vi "Turn filter wheel by angle.vi"(8 "Clockwise?":bool=TRUE, 9 "Error In":errorcluster, 11 "Angle (degrees)":dbl=50.5244026184082) -> (0 "error out":errorcluster, 2 "Enable Channel out":u8=11, 3 "Serial Port out":refnum<visa-resource-name>="COM3")   [LabVIEW 2011]
uses:
  <vilib>/MakerHub/LINX/Public/Peripherals/Digital/Digital Write 1 Chan.vi
  <vilib>/MakerHub/LINX/LMH-LINX.lvlib
panel:
  in  "Enable Channel":u8=11
  in  "Direction Channel":u8=8
  in  "Step Channel":u8=9
  in  "Serial Port":refnum<visa-resource-name>="COM6"
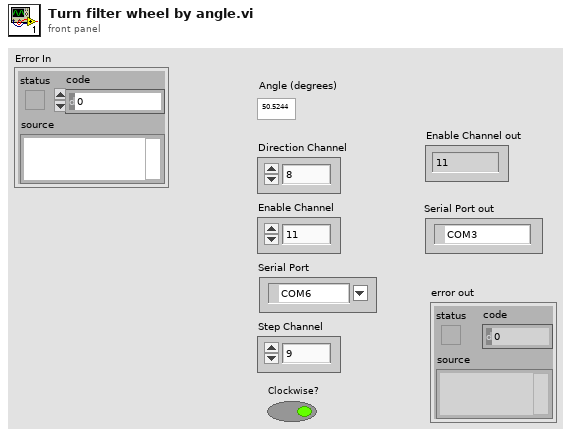
[diagram p1: front panel]
types:
  T1 = typedef "LMH-LINX.lvlib/LINX Ref.ctl" = cluster{"Platform":T2, "Interface":T3, "LINX Device Config":T4}
  T2 = typedef "LMH-LINX.lvlib/Platform.ctl" = enum16{"LINX", "myRIO"}
  T3 = typedef "LMH-LINX.lvlib/Interface.ctl" = enum16{"Serial", "TCP"}
  T4 = typedef "LMH-LINX.lvlib/Device.lvlib/LINX Device Config.ctl" = cluster{"Interface":T3, "COM Port":refnum<visa-resource-name>, "TCP Configuration":T5, "Device Family":u8, "Device ID":u8, "Device Name":string, "TCP Ref":refnum<k5>, "Channels":T6}
  T5 = typedef "LMH-LINX.lvlib/Device.lvlib/TCP Config.ctl" = cluster{"IP Address":string, "Port":u16}
  T6 = typedef "LMH-LINX.lvlib/Channels.ctl" = cluster{"DI":u8[], "DO":u8[], "AI":u8[], "AO":u8[], "PWM":u8[], "QE":u8[], "UART":u8[], "I2C 2":u8[], "SPI":u8[], "CAN":u8[], "Servo":u8[], "AI Ref (V)":dbl, "AO Ref (V)":dbl, "AO Resolution (Bits)":u8}
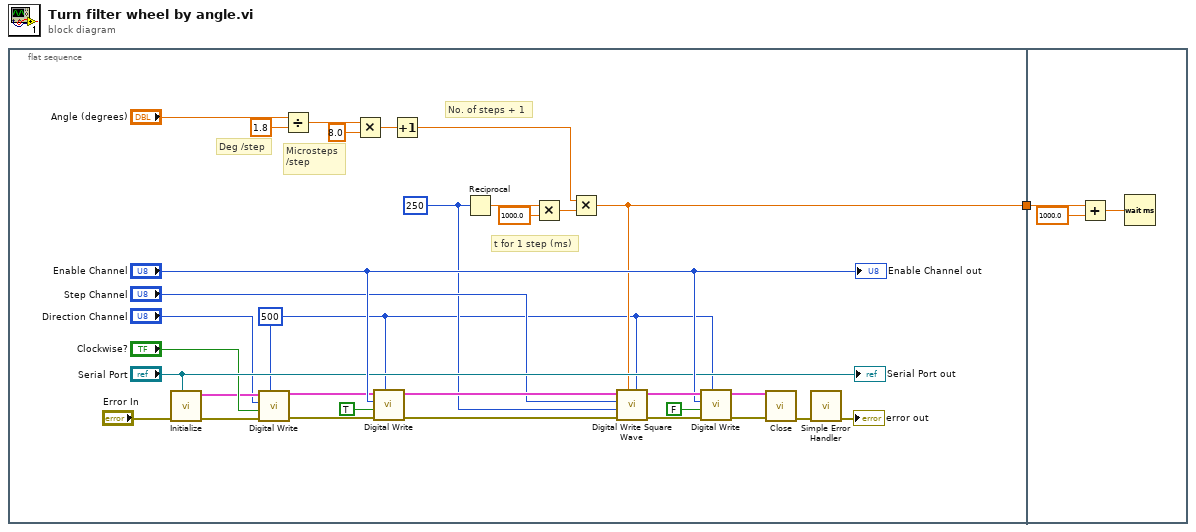
[diagram p0: block diagram]
diagram:
  n1 = flat-sequence {
    tunnel: [w3] -> w1
    tunnel: w1 -> [w35]
    frame #0 {
      w2 = 500 ("Timeout (100 ms)")
      w10 = u32 250 ("Frequency (Hz)")
      # "t for 1 step (ms)"
      # "No. of steps + 1"
      # "Microsteps\n/step"
      # "Deg /step"
      n2 = call <vilib>:"Initialize.vi"("Serial Port"="Serial Port", "Error In"="Error In") -> ("Error Out"=w22:errorcluster, "LINX Ref"=w23:T1)  [unwired: 7 in, 1 out]
      n3 = call-poly <vilib>:"Digital Write.vi"("Timeout (100 ms)"=w2, "Error In"=w22, "Output Value"="Clockwise?", "DO Channel"="Direction Channel", "LINX Resource"=w23) -> ("Error Out"=w15:errorcluster, "LINX Resource"=w16:T1)  [unwired: 5 in]
      n4 = Divide(x="Angle (degrees)", y=1.8) -> (x/y=w12:dbl)
      n5 = Multiply(x=w12, y=8.0) -> (x*y=w6:dbl)
      n6 = call-poly <vilib>:"Digital Write.vi"("Timeout (100 ms)"=w2, "Error In"=w15, "Output Value"=TRUE ("LED Value"), "DO Channel"="Enable Channel", "LINX Resource"=w16) -> ("Error Out"=w18:errorcluster, "LINX Resource"=w19:T1)  [unwired: 5 in]
      n7 = Increment(x=w6) -> (x+1=w5:dbl)
      n8 = Reciprocal(x=w10) -> (1/x=w9:dbl)
      n9 = Multiply(x=w9, y=1000.0) -> (x*y=w7:dbl)
      n10 = Multiply(x=w5, y=w7) -> (x*y=w3:dbl)
      n11 = call <vilib>:"Digital Write Square Wave.vi"("Timeout (100 ms)"=w2, "Duration (ms)"=w3, "Error In"=w18, "Frequency (Hz)"=w10, "Channel"="Step Channel", "LINX Resource"=w19) -> ("Error Out"=w30:errorcluster, "LINX Resource"=w31:T1)  [unwired: 4 in]
      n12 = call-poly <vilib>:"Digital Write.vi"("Timeout (100 ms)"=w2, "Error In"=w30, "Output Value"=FALSE ("LED Value"), "DO Channel"="Enable Channel", "LINX Resource"=w31) -> ("Error Out"=w27:errorcluster, "LINX Resource"=w28:T1)  [unwired: 5 in]
      n13 = call <vilib>:"Close.vi"("Error In"=w27, "LINX Resource"=w28) -> ("Error Out"=w33:errorcluster)  [unwired: 8 in, 1 out]
      n14 = call <vilib>:"Simple Error Handler.vi"("error in (no error)"=w33) -> ("error out"=→"error out":errorcluster)  [unwired: 4 in, 4 out]
      "Serial Port out" <- "Serial Port"
      "Enable Channel out" <- "Enable Channel"
    }
    frame #1 {
      n15 = Add(x=w35, y=1000.0) -> (x+y=w34:dbl)
      n16 = Wait (ms)(milliseconds to wait=w34) -> ()  [unwired: 1 out]
    }
  }
